vi "Guardar datos de Amplitud y Tiempo.vi"(0 "path":path, 3 "Datos experimento":string[][](array[string]), 4 "column headers":string[](array[string])=["Tiempo", "Amplitud"]) -> ()   [LabVIEW 2024]
uses:
  <vilib>/addons/_office/excel.llb/Excel Easy Table (str).vi
  <vilib>/Utility/NIReport.llb/NI_report.lvclass
  <vilib>/Utility/NIReport.llb/Excel/NI_Excel.lvclass
  <vilib>/addons/_office/NI_ReportGenerationToolkit.lvlib
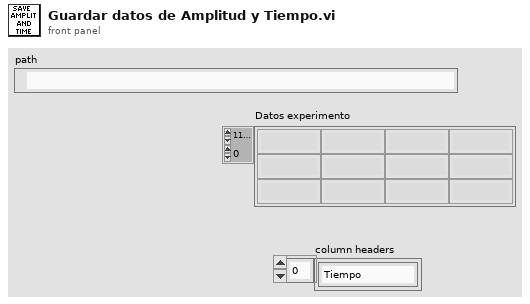
[diagram p1: front panel]
types:
  T1 = enum16{"Standard Report", "HTML", "Word", "Excel"}
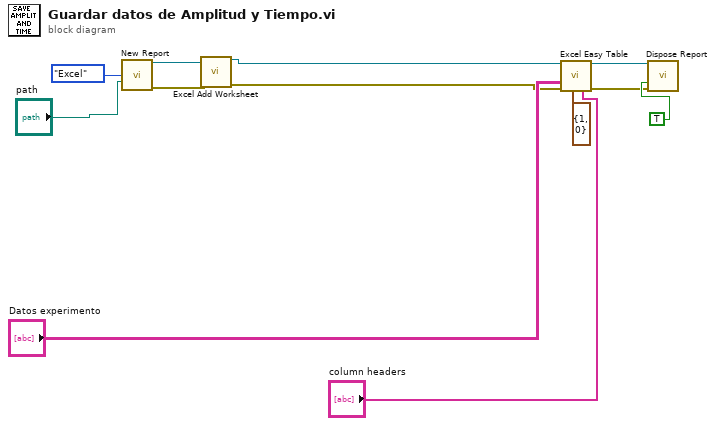
[diagram p0: block diagram]
diagram:
  n1 = call <vilib>:"New Report.vi"("report type"=T1."Excel", "template (empty)"="path") -> ("report out"=w11:refnum<class "NI_report.lvclass">, "error out"=w10:errorcluster)  [unwired: 12 in]
  n2 = call <vilib>:"Excel Add Worksheet.vi"("report in"=w11, "error in (no error)"=w10) -> ("report out"=w3:refnum<class "NI_report.lvclass">, "error out"=w2:errorcluster)  [unwired: 12 in]
  n3 = call-poly <vilib>:"Excel Easy Table.vi"("report in"=w3, "start (0, 0)"=cluster{"row":i32, "column":i32} {"row"=1, "column"=0}, "text data"="Datos experimento", "error in (no error)"=w2, "column headers"="column headers") -> ("report out"=w7:refnum<class "NI_report.lvclass">, "error out"=w1:errorcluster)  [unwired: 6 in, 3 out]
  n4 = call-dynamic "Dispose Report.vi"("report in"=w7, "save changes? (F)"=TRUE ("close report? (T)"), "error in (no error)"=w1) -> ()  [unwired: 12 in, 1 out]
